vi "FunctionGeneratorMain.vi"() -> ()   [LabVIEW 2020]
uses:
  FunctionGenerator.lvclass
panel:
  in  "error in (no error)":errorcluster
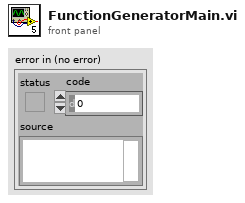
[diagram p1: front panel]
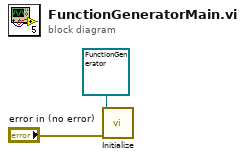
[diagram p0: block diagram]
diagram:
  n1 = call-dynamic "Initialize.vi"("error in (no error)"="error in (no error)", "FunctionGenerator in"=refnum<class "FunctionGenerator.lvclass"> refnum) -> ()  [unwired: 8 in, 2 out]
